vi "Verify.VITester.vi"(8 "error in (no error)":errorcluster, 10 "Test Data":string, 11 "TestCase in":refnum<class "TestCase.lvclass">) -> (0 "error out":errorcluster, 3 "TestCase out":refnum<class "TestCase.lvclass">)   [LabVIEW 2020]
uses:
  <vilib>/addons/_JKI Toolkits/VI Tester/TestCase.llb/TestCase.lvclass
  <vilib>/SAS/Approval Tests/lib_Approval Tests.lvlib
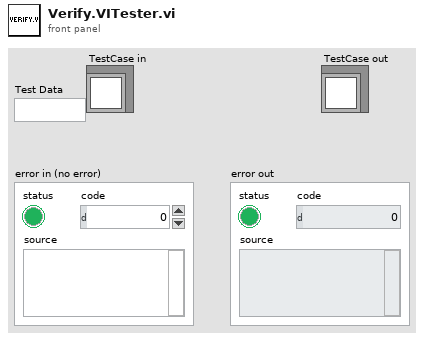
[diagram p1: front panel]
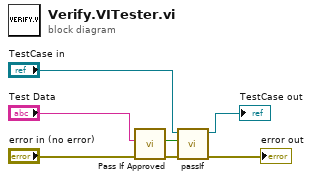
[diagram p0: block diagram]
diagram:
  n1 = call <vilib>:"Pass If Approved.vi"("error in"="error in (no error)", "Test Data"="Test Data") -> ("error out"=w5:errorcluster, "Passed?"=w3:bool)  [unwired: 7 in, 1 out]
  n2 = call-dynamic "passIf.vi"("error in (no error)"=w5, "pass"=w3, "TestCase in"="TestCase in") -> ("error out"=→"error out":errorcluster, "TestCase out"=→"TestCase out":refnum<class "TestCase.lvclass">)  [unwired: 7 in]
